vi "IT8800-Configure Input.vi"(8 "error in":errorcluster, 9 "Enable Input Short":bool, 10 "Enable Input":bool, 11 "IT8800 Setting In In":T1={"VISA Resource Name"="", "Baud Rate"=19200, "Stop Bits"=20, "Wait For Read(ms)"=0, "Interface Type"=enum."VXI", "Limits"=[]} {"Stop Bits" items=["1.0"=10, "2.0"=20]; "Baud Rate" items=["2400"=2400, "4800"=4800, "9600"=9600, "19200"=19200]}) -> (0 "error out":errorcluster, 3 "IT8800 Setting In Out":T1={"VISA Resource Name"="", "Baud Rate"=19200, "Stop Bits"=20, "Wait For Read(ms)"=0, "Interface Type"=enum."VXI", "Limits"=[]} {"Stop Bits" items=["1.0"=10, "2.0"=20]; "Baud Rate" items=["2400"=2400, "4800"=4800, "9600"=9600, "19200"=19200]})   [LabVIEW 2018]
doc: "Configures the input state and the input short to either on or off."
uses:
  Data Def/IT8800-Setting.ctl
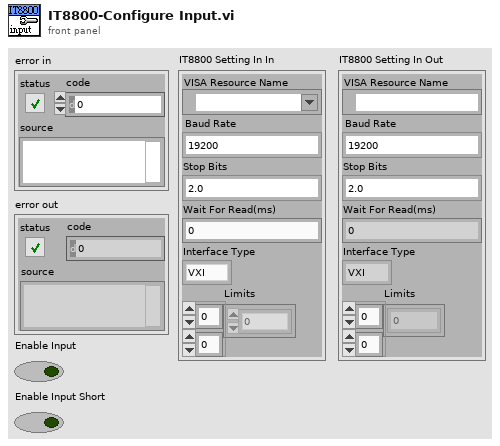
[diagram p1: front panel]
types:
  T1 = typedef "IT8800-Setting.ctl" = cluster{"VISA Resource Name":refnum<visa-resource-name>, "Baud Rate":u32, "Stop Bits":u16, "Wait For Read(ms)":u32, "Interface Type":enum16{"Unknow", "GPIB", "VXI", "GPIB-VXI", "Serial", "PXI", "TCPIP", "USB", "FireWire"}, "Limits":dbl[][]}
  T2 = typedef "IT8800-Operation Mode.ctl" = enum16{"Constant Current(CC)", "Constant Voltage(CV)", "Constant Power(CP)", "Constant Resistance(CR)"}
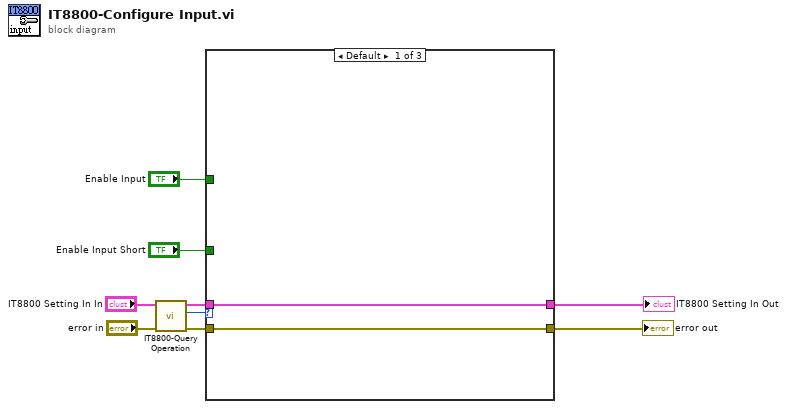
[diagram p0: block diagram]
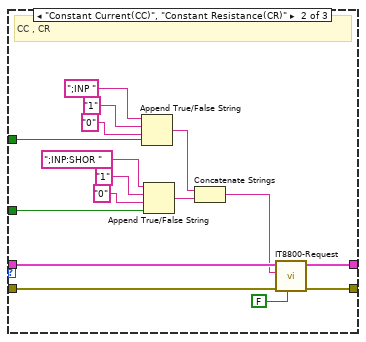
[diagram p2: hidden frame]
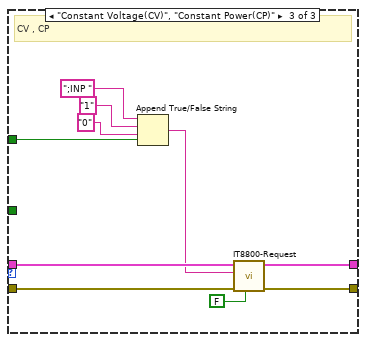
[diagram p3: hidden frame]
diagram:
  n1 = call "IT8800-Query Operation.vi"("error in"="error in", "IT8800 Setting In In"="IT8800 Setting In In") -> ("error out"=w3:errorcluster, "Operation Mode"=w2:T2, "IT8800 Setting In Out"=w4:T1)  [unwired: 7 in]
  n2 = case shown="Default" w2 {
    tunnel: w4 -> [w11 w16 w30]
    tunnel: w3 -> [w10 w17 w33]
    tunnel: "Enable Input" -> [_ w21 w34]
    tunnel: "Enable Input Short" -> [_ w20 _]
    tunnel: [w10 w14 w32] -> w7
    tunnel: [w11 w15 w31] -> w6
    frame Default {
    }
    frame "Constant Current(CC)", "Constant Resistance(CR)" {
      # "CC , CR"
      n3 = Append True/False String(1:w21, 2:"0" ("false string"), 3:"1" ("true string"), 4:";INP " ("string (\"\")")) -> (0:w18:string)
      n4 = Append True/False String(1:w20, 2:"0" ("false string"), 3:"1" ("true string"), 4:";INP:SHOR " ("string (\"\")")) -> (0:w19:string)
      n5 = Concatenate Strings(w18, w19) -> (w13:string)
      n6 = call "IT8800-Request.vi"("Response?"=FALSE, "error in"=w17, "Command"=w13, "IT8800 Setting In In"=w16) -> ("error out"=w14:errorcluster, "IT8800 Setting In Out"=w15:T1)  [unwired: 5 in, 1 out]
    }
    frame "Constant Voltage(CV)", "Constant Power(CP)" {
      # "CV , CP"
      n7 = Append True/False String(1:w34, 2:"0" ("false string"), 3:"1" ("true string"), 4:";INP " ("string (\"\")")) -> (0:w29:string)
      n8 = call "IT8800-Request.vi"("Response?"=FALSE, "error in"=w33, "Command"=w29, "IT8800 Setting In In"=w30) -> ("error out"=w32:errorcluster, "IT8800 Setting In Out"=w31:T1)  [unwired: 5 in, 1 out]
    }
  }
  "error out" <- w7
  "IT8800 Setting In Out" <- w6
